vi "clean_esp_html.vi"(0 "Body":string) -> (1 "Cleaned Body":string, 2 "appended array":string[](array[string]))   [LabVIEW 2017]
uses:
  <vilib>/regexp/Match Regular Expression.xnode
panel:
  out "Iteration":i32
  out "after match":string
  out "whole match":string
  out "before match":string
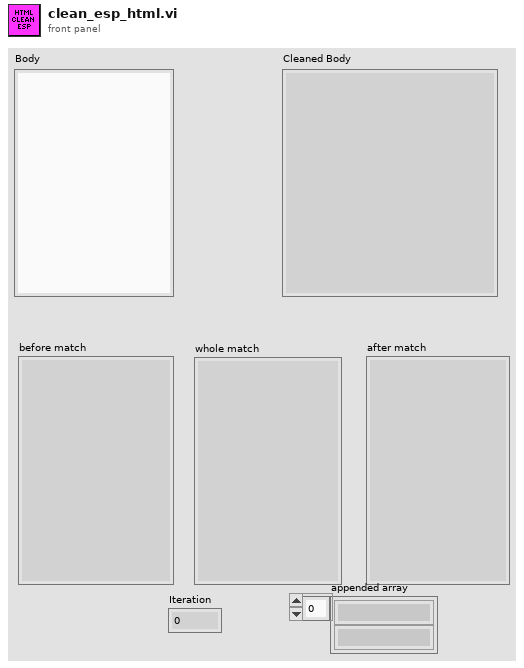
[diagram p1: front panel]
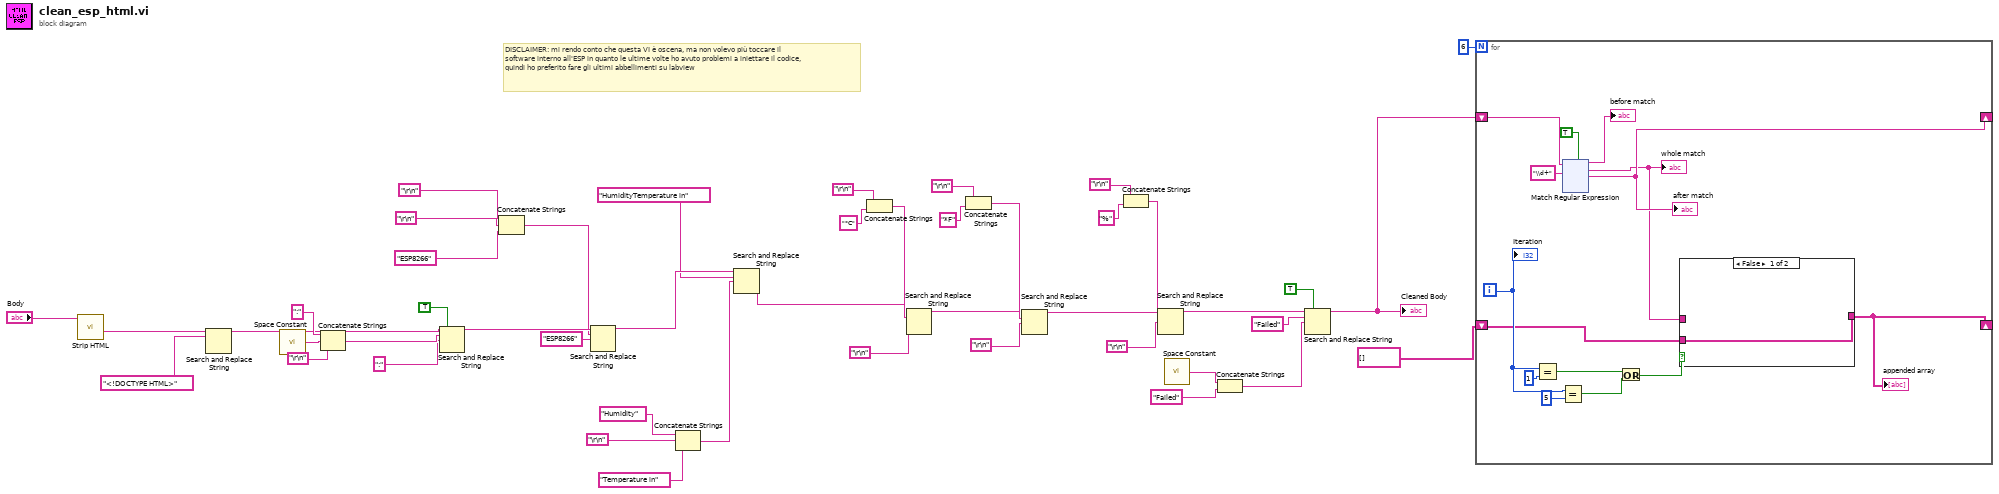
[diagram p0: block diagram]
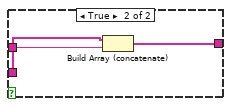
[diagram p2: hidden frame]
diagram:
  # "DISCLAIMER: mi rendo conto che questa VI è oscena, ma non volevo più toccare il software interno all'ESP in quanto le ultime volte ho avuto problemi a iniettare il codice, quindi ho preferito fare gli ultimi abbellimenti su labview"
  n1 = call "Strip HTML.vi"("HTML String"="Body") -> ("HTML Stripped String"=w46:string)  [unwired: 6 in, 4 out]
  n2 = Search and Replace String(input string=w46, search string="<!DOCTYPE HTML>") -> (result string=w39:string)  [unwired: 6 in, 3 out]
  n3 = call <vilib>:"Space Constant.vi"() -> ("String"=w43:string)
  n4 = Concatenate Strings(":" ("string"), w43, "\r\n") -> (w41:string)
  n5 = Search and Replace String(replace all?=TRUE ("replace all? (F)"), input string=w39, search string=w41, replace string=":" ("replace string (\"\")")) -> (result string=w34:string)  [unwired: 4 in, 3 out]
  n6 = Concatenate Strings("\r\n", "\r\n", "ESP8266") -> (w33:string)
  n7 = Search and Replace String(input string=w34, search string=w33, replace string="ESP8266" ("replace string (\"\")")) -> (result string=w31:string)  [unwired: 5 in, 3 out]
  n8 = Concatenate Strings("Humidity" ("string"), "\r\n", "Temperature in" ("string")) -> (w12:string)
  n9 = Search and Replace String(input string=w31, search string="HumidityTemperature in", replace string=w12) -> (result string=w11:string)  [unwired: 5 in, 3 out]
  n10 = Concatenate Strings("\r\n", "*C" ("string")) -> (w20:string)
  n11 = Search and Replace String(input string=w11, search string=w20, replace string="\r\n") -> (result string=w17:string)  [unwired: 5 in, 3 out]
  n12 = Concatenate Strings("\r\n", "*F" ("string")) -> (w19:string)
  n13 = Search and Replace String(input string=w17, search string=w19, replace string="\r\n") -> (result string=w16:string)  [unwired: 5 in, 3 out]
  n14 = Concatenate Strings("\r\n", "%" ("string")) -> (w18:string)
  n15 = Search and Replace String(input string=w16, search string=w18, replace string="\r\n") -> (result string=w9:string)  [unwired: 5 in, 3 out]
  n16 = call <vilib>:"Space Constant.vi"() -> ("String"=w6:string)
  n17 = Concatenate Strings(w6, "Failed" ("string")) -> (w7:string)
  n18 = Search and Replace String(replace all?=TRUE ("replace all? (F)"), input string=w9, search string="Failed", replace string=w7) -> (result string=w2:string)  [unwired: 4 in, 3 out]
  "Cleaned Body" <- w2
  n19 = for {
    N: 6 -> [_]
    shift-right: [w56] -> _
    shift-left: w2 -> [w57]
    shift-right: [w48] -> _
    shift-left: string[] [] -> [w50]
    i -> [w55]
    n20 = Equal?(x=w55, y=1) -> (x = y?=w52:bool)
    n21 = Equal?(x=w55, y=5) -> (x = y?=w51:bool)
    n22 = xnode "Match Regular Expression"("input string"=w57, "regular expression"="\\d+", "multiline? (F)"=TRUE) -> ("before match"=→"before match":string, "whole match"=w49:string, "after match"=w56:string)  [unwired: 3 in, 2 out]
    "whole match" <- w49
    "after match" <- w56
    n23 = Or(x=w52, y=w51) -> (x .or. y?=w47:bool)
    n24 = case shown="False" w47 {
      tunnel: w50 -> [w61 w64]
      tunnel: w49 -> [_ w63]
      tunnel: [w61 w62] -> w48
      frame False {
      }
      frame True {
        n25 = Build Array (concatenate)(w64, w63) -> (w62:string[])
      }
    }
    "appended array" <- w48
    "Iteration" <- w55
  }
